vi "pp2_log_sessionParameters.vi"(10 "refnum in":refnum<file>, 11 "Session parameters":T1={"Log File Directory Root"=path "C:/test", "Habit tr0 (s)"=180, "ITI max\n(s)"=25, "ITI min\n(s)"=15, "Tone repeat (ms)"=0, "Jump time\n(s)"=4, "Subject Name"="SPP030", "Run"=FALSE, "Start trial"=0, "Stay \n(s)"=5, "Log File Directory"=path "", "Shock \ndur (s)"=6, "Pre click \n(V)"=1.0, "Click\ndel (s)"=6.0} {"Click\ndel (s)" min=0.0 step=1.0; "Pre click \n(V)" min=0.0 step=1.0; "Shock \ndur (s)" min=0 step=1; "Stay \n(s)" min=0 step=1; "Start trial" step=1; "Jump time\n(s)" min=0 step=1; "Tone repeat (ms)" min=0 step=1; "ITI min\n(s)" min=0 step=1; "ITI max\n(s)" min=0 step=1; "Habit tr0 (s)" min=0 step=1}) -> (2 "refnum out":refnum<file>)   [LabVIEW 2013]
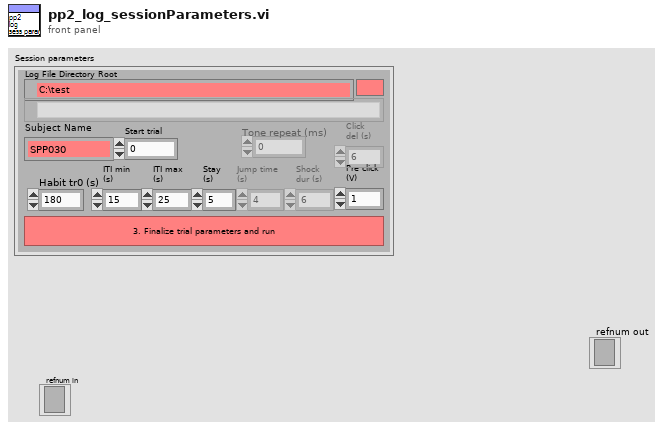
[diagram p1: front panel]
types:
  T1 = cluster{"Log File Directory Root":path, "Habit tr0 (s)":i32, "ITI max\n(s)":i32, "ITI min\n(s)":i32, "Tone repeat (ms)":i32, "Jump time\n(s)":i32, "Subject Name":string, "Run":bool, "Start trial":u16, "Stay \n(s)":i32, "Log File Directory":path, "Shock \ndur (s)":i32, "Pre click \n(V)":dbl, "Click\ndel (s)":dbl}
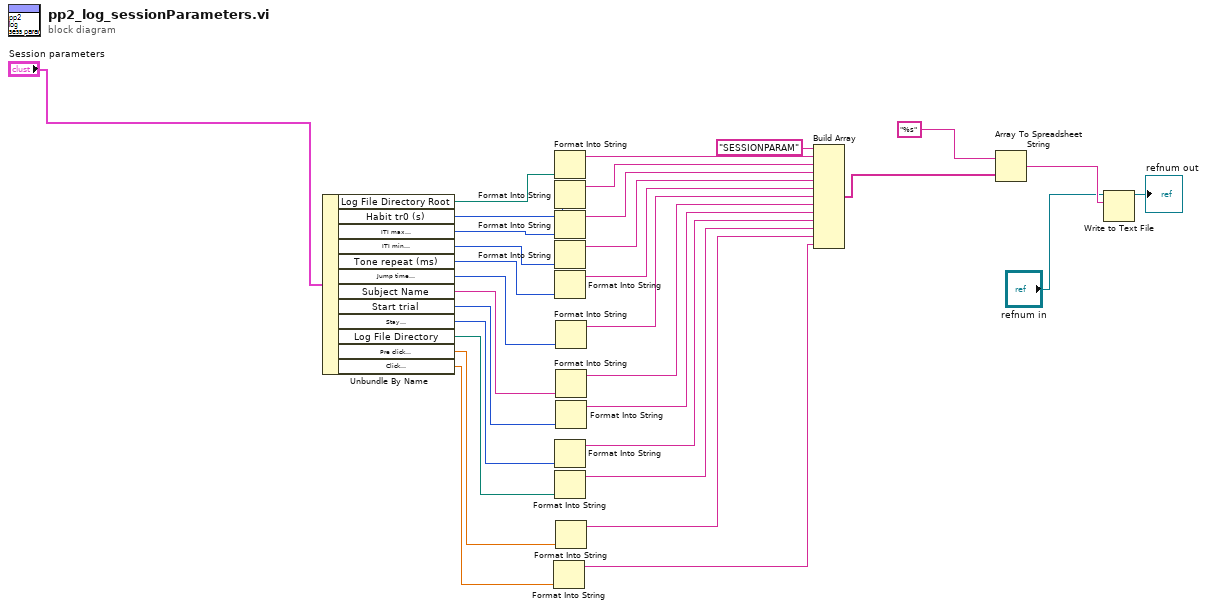
[diagram p0: block diagram]
diagram:
  n1 = Unbundle By Name("Session parameters") -> ("Log File Directory Root"=w31:path, "Habit tr0 (s)"=w28:i32, "ITI max\n(s)"=w27:i32, "ITI min\n(s)"=w26:i32, "Tone repeat (ms)"=w25:i32, "Jump time\n(s)"=w24:i32, "Subject Name"=w18:string, "Start trial"=w17:u16, "Stay \n(s)"=w16:i32, "Log File Directory"=w15:path, "Pre click \n(V)"=w14:dbl, "Click\ndel (s)"=w3:dbl)
  n2 = Format Into String(w3) -> (resulting string=w2:string)  [unwired: 3 in, 1 out]
  n3 = Format Into String(w31) -> (resulting string=w30:string)  [unwired: 3 in, 1 out]
  n4 = Format Into String(w28) -> (resulting string=w23:string)  [unwired: 3 in, 1 out]
  n5 = Format Into String(w27) -> (resulting string=w22:string)  [unwired: 3 in, 1 out]
  n6 = Format Into String(w26) -> (resulting string=w21:string)  [unwired: 3 in, 1 out]
  n7 = Format Into String(w25) -> (resulting string=w20:string)  [unwired: 3 in, 1 out]
  n8 = Format Into String(w16) -> (resulting string=w11:string)  [unwired: 3 in, 1 out]
  n9 = Format Into String(w15) -> (resulting string=w10:string)  [unwired: 3 in, 1 out]
  n10 = Format Into String(w24) -> (resulting string=w19:string)  [unwired: 3 in, 1 out]
  n11 = Format Into String(w18) -> (resulting string=w13:string)  [unwired: 3 in, 1 out]
  n12 = Format Into String(w17) -> (resulting string=w12:string)  [unwired: 3 in, 1 out]
  n13 = Format Into String(w14) -> (resulting string=w9:string)  [unwired: 3 in, 1 out]
  n14 = Build Array("SESSIONPARAM" ("element"), w30, w23, w22, w21, w20, w19, w13, w12, w11, w10, w9, w2) -> (w6:string[])
  n15 = Array To Spreadsheet String(array=w6, 3:"%s" ("format string")) -> (spreadsheet string=w7:string)  [unwired: 1 in]
  n16 = Write to Text File(file (use dialog)="refnum in", text=w7) -> (refnum out=→"refnum out":refnum<file>)  [unwired: 2 in, 2 out]
